vi "Stop data taking procedure (SubVI).vi"(2 "error in (no error)":errorcluster, 3 "stop":refnum<vi>, 4 "is_stopping?":refnum<vi>, 5 "Queue in":refnum<queue>) -> (0 "error out":errorcluster)   [LabVIEW 2016]
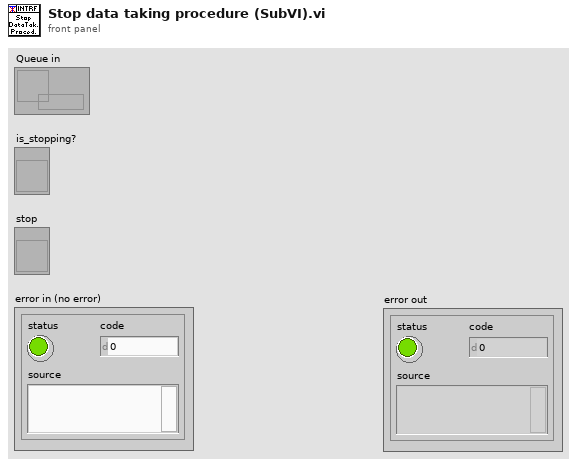
[diagram p1: front panel]
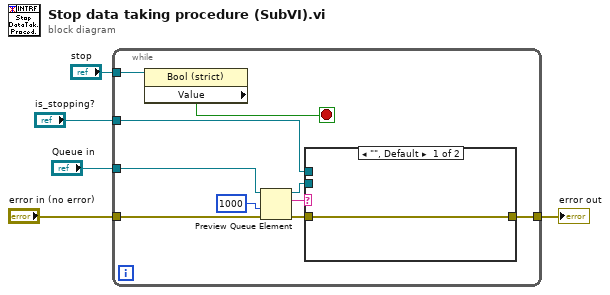
[diagram p0: block diagram]
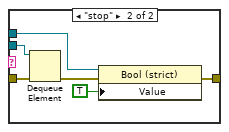
[diagram p2: hidden frame]
diagram:
  n1 = while {
    tunnel: "Queue in" -> [w15]
    tunnel: "error in (no error)" -> [w14]
    tunnel: "stop" -> [w9]
    tunnel: "is_stopping?" -> [w7]
    tunnel: [w6] -> w1
    stop <- w10 stop-if-true
    n2 = property class="Bool (strict)"(reference=w9) -> ("Value"=w10:bool)  [unwired: 1 in, 2 out]
    n3 = Preview Queue Element(queue=w15, timeout in ms (-1)=1000, error in (no error)=w14) -> (queue out=w11:refnum<queue>, element=w13:string, error out=w12:errorcluster)  [unwired: 1 out]
    n4 = case shown="\"\", Default" w13 {
      tunnel: w12 -> [w16 w21]
      tunnel: w11 -> [_ w22]
      tunnel: w7 -> [_ w19]
      tunnel: [w16 w17] -> w6
      frame "", Default {
      }
      frame "stop" {
        n5 = Dequeue Element(queue=w22, error in (no error)=w21) -> (error out=w18:errorcluster)  [unwired: 1 in, 3 out]
        n6 = property class="Bool (strict)"(reference=w19, error in=w18, "Value"=TRUE) -> (error out=w17:errorcluster)  [unwired: 1 out]
      }
    }
  }
  "error out" <- w1
